vi "_30_Sample_qsns_9[6].vi"() -> ()   [LabVIEW 2020]
panel:
  out "x-y":i32[](array[numeric])
  out "size(s)":i32[](array[numeric])
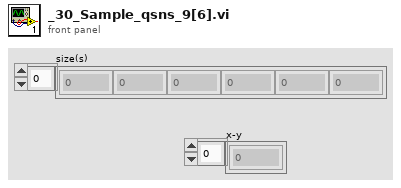
[diagram p1: front panel]
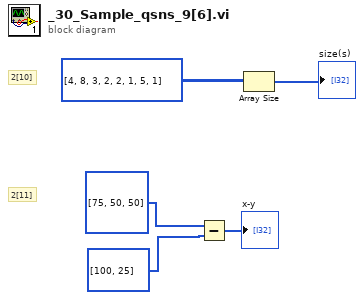
[diagram p0: block diagram]
diagram:
  # "2[11]"
  # "2[10]"
  n1 = Subtract(x=i32[] [75, 50, 50], y=i32[] [100, 25]) -> (x-y=→"x-y":i32[])
  n2 = Array Size(array=i32[][] [[4, 8, 3, 2], [2, 1, 5, 1]]) -> (size(s)=→"size(s)":i32[])
